vi "Locate Kernel in Path.vi"(8 "error in (no error)":errorcluster, 11 "object in":refnum<class "JuPyter_Client.lvclass">) -> (0 "error out":errorcluster, 2 "Path to ipython":path, 3 "object out":refnum<class "JuPyter_Client.lvclass">)   [LabVIEW 2018, in "JuPyter_Client.lvclass"]
doc: "Look at the OS environment path variable for an ipython.exe"
uses:
  JuPyter_Client.lvclass
  <vilib>/registry/registry.llb/Read Registry Value Simple STR.vi
  <vilib>/registry/registry.llb/Registry SAM.ctl
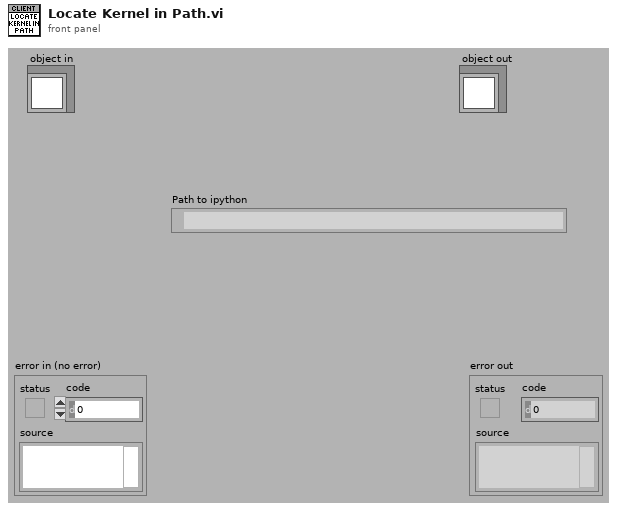
[diagram p1: front panel]
types:
  T1 = typedef "Registry SAM.ctl" = enum32{"KEY_QUERY_VALUE", "KEY_SET_VALUE", "KEY_CREATE_SUB_KEY", "KEY_ENUMERATE_SUB_KEYS", "KEY_NOTIFY", "KEY_CREATE_LINK", "KEY_READ", "KEY_WRITE", "KEY_ALL_ACCESS", "KEY_READ | KEY_WRITE"}
  T2 = typedef "Registry RtKey.ctl" = enum32{"HKEY_CLASSES_ROOT", "HKEY_CURRENT_USER", "HKEY_LOCAL_MACHINE", "HKEY_USERS", "HKEY_PERFORMANCE_DATA", "HKEY_CURRENT_CONFIG", "HKEY_DYN_DATA"}
  T3 = typedef "Registry refnum.ctl" = refnum<k1>
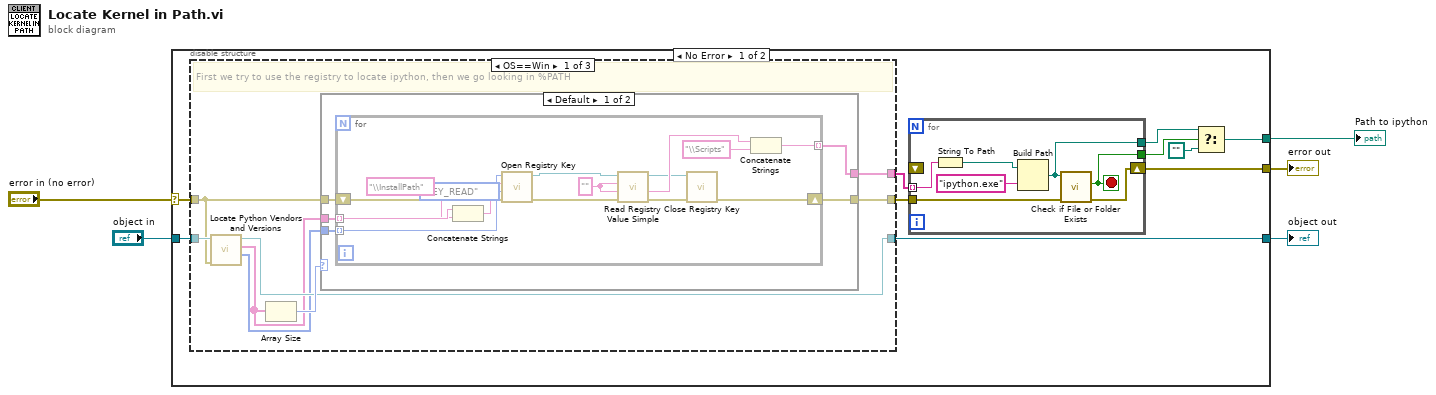
[diagram p0: block diagram]
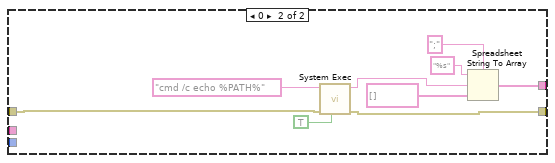
[diagram p2: hidden frame]
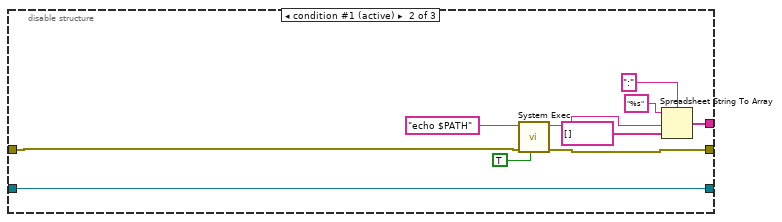
[diagram p3: hidden frame]
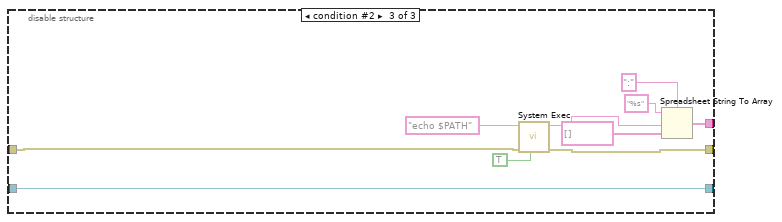
[diagram p4: hidden frame]
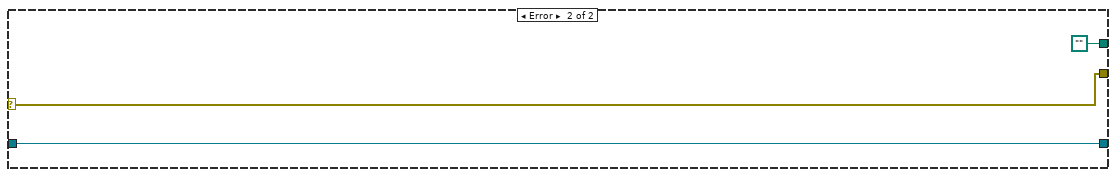
[diagram p5: hidden frame]
diagram:
  n1 = case shown="No Error" "error in (no error)" {
    selector: "error in (no error)" -> [w15 w82]
    tunnel: [w8 w82] -> w4
    tunnel: [w6 w81] -> w2
    tunnel: "object in" -> [w7 w81]
    tunnel: [w10 path ""] -> w1
    frame No Error {
      n2 = disable-structure shown="OS==Win" {
        disable-tunnel: w15 -> [w27 w67 w77]
        disable-tunnel: [w30 w66 w76] -> w9
        disable-tunnel: [w29 w62 w72] -> w14
        disable-tunnel: [w25 w60 w70] -> w6
        disable-tunnel: w7 -> [w28 w60 w70]
        frame condition #0 {
          # "First we try to use the registry to locate ipython, then we go looking in %PATH"
          n3 = call "Locate Python Vendors and Versions.vi"("error in (no error)"=w27, "object in"=w28) -> ("Hives"=w23:T2[], "Python Sub keys"=w24:string[], "object out"=w25:refnum<class "JuPyter_Client.lvclass">)  [unwired: 6 in, 1 out]
          n4 = Array Size(array=w24) -> (size(s)=w26:i32)
          n5 = case shown="Default" w26 {
            tunnel: [w31 w57] -> w30
            tunnel: [w33 w53] -> w29
            tunnel: w27 -> [w32 w51]
            tunnel: w24 -> [w35 _]
            tunnel: w23 -> [w34 _]
            frame Default {
              n6 = for {
                tunnel: w35 -> [w49] mode=indexing
                tunnel: w34 -> [w50] mode=indexing
                tunnel: [w41] -> w33 mode=indexing
                shift-right: [w37] -> w31
                shift-left: w32 -> [w38]
                w44 = "" ("value")
                n7 = Concatenate Strings(w49, "\\InstallPath" ("string")) -> (w48:string)
                n8 = call <vilib>:"Open Registry Key.vi"("error in (no error)"=w38, "security access mask (KEY_READ | KEY_WRITE)"=Registry_SAM."KEY_READ", "subkey"=w48, "root key (HKEY_LOCAL_MACHINE)"=w50) -> ("error out"=w46:errorcluster, "refnum out"=w45:T3)  [unwired: 6 in]
                n9 = call-poly <vilib>:"Read Registry Value Simple.vi"("error in (no error)"=w46, "default data"=w44, "value"=w44, "refnum"=w45) -> ("error out"=w40:errorcluster, "String/Binary data"=w43:string, "refnum out"=w39:T3)  [unwired: 2 in, 1 out]
                n10 = call <vilib>:"Close Registry Key.vi"("error in (no error)"=w40, "refnum"=w39) -> ("error out"=w37:errorcluster)  [unwired: 5 in]
                n11 = Concatenate Strings(w43, "\\Scripts" ("string")) -> (w41:string)
              }
            }
            frame 0 {
              n12 = call <vilib>:"System Exec.vi"("run minimized? (F)"=TRUE, "error in (no error)"=w51, "command line"="cmd /c echo %PATH%") -> ("error out"=w57:errorcluster, "standard output"=w55:string)  [unwired: 5 in, 2 out]
              n13 = Spreadsheet String To Array(delimiter (Tab)=";", format string="%s", spreadsheet string=w55, array type (2D Dbl)=string[] []) -> (array=w53:string[])
            }
          }
        }
        frame condition #1 (active) {
          n14 = call <vilib>:"System Exec.vi"("run minimized? (F)"=TRUE, "error in (no error)"=w67, "command line"="echo $PATH") -> ("error out"=w66:errorcluster, "standard output"=w64:string)  [unwired: 5 in, 2 out]
          n15 = Spreadsheet String To Array(delimiter (Tab)=":", format string="%s", spreadsheet string=w64, array type (2D Dbl)=string[] []) -> (array=w62:string[])
        }
        frame condition #2 {
          n16 = call <vilib>:"System Exec.vi"("run minimized? (F)"=TRUE, "error in (no error)"=w77, "command line"="echo $PATH") -> ("error out"=w76:errorcluster, "standard output"=w74:string)  [unwired: 5 in, 2 out]
          n17 = Spreadsheet String To Array(delimiter (Tab)=":", format string="%s", spreadsheet string=w74, array type (2D Dbl)=string[] []) -> (array=w72:string[])
        }
      }
      n18 = for {
        tunnel: w14 -> [w22] mode=indexing
        tunnel: [w19] -> w12
        tunnel: [w18] -> w13
        tunnel: w9 -> [w17]
        shift-right: [w16] -> w8
        shift-left: _ -> [_]
        stop <- w18 stop-if-true
        n19 = String To Path(string=w22) -> (path=w21:path)
        n20 = Build Path(base path=w21, name or relative path="ipython.exe") -> (appended path=w19:path)
        n21 = call <vilib>:"Check if File or Folder Exists.vi"("error in (no error)"=w17, "path"=w19) -> ("error out"=w16:errorcluster, "file or folder exists?"=w18:bool)  [unwired: 7 in, 1 out]
      }
      n22 = Select(t=w12, s=w13, f=path "") -> (s? t:f=w10:path)
    }
    frame Error {
    }
  }
  "error out" <- w4
  "object out" <- w2
  "Path to ipython" <- w1
